vi "date_string_concatenation_log_record.vi"(10 "Cluster":T1, 11 "st_LogEvent":string) -> (3 "st_logrecord":string)   [LabVIEW 2026]
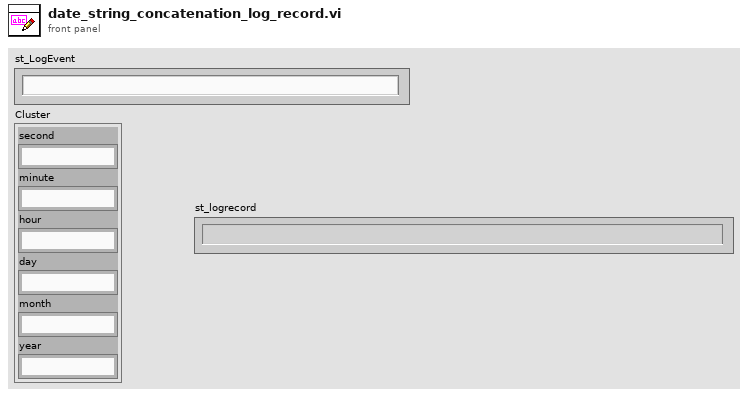
[diagram p1: front panel]
types:
  T1 = cluster{"second":string, "minute":string, "hour":string, "day":string, "month":string, "year":string}
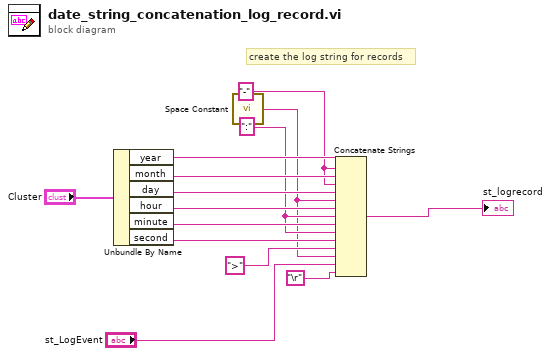
[diagram p0: block diagram]
diagram:
  w4 = ":"
  w11 = "-"
  # "create the log string for records"
  n1 = Unbundle By Name("Cluster") -> ("year"=w13:string, "month"=w12:string, "day"=w10:string, "hour"=w9:string, "minute"=w8:string, "second"=w7:string)
  n2 = call <vilib>:"Space Constant.vi"() -> ("String"=w2:string)
  n3 = Concatenate Strings(w13, w11, w12, w11, w10, w2, w9, w4, w8, w4, w7, ">", w2, "st_LogEvent", "\r") -> (→"st_logrecord":string)
